vi "Actor Core.vi"(8 "error in":errorcluster, 11 "GObject View in":refnum<class "GObject View.lvclass">) -> (0 "error out":errorcluster, 3 "Actor out":refnum<class "Actor.lvclass">)   [LabVIEW 2013, in "SET Project Editor.lvlib" / "GObject View.lvclass"]
doc: "(<B>Filename</B>: Actor Framework.lvlib:Actor.lvclass:Actor Core.vi)\n\nReceives messages to the actor, reacts to them, and initiates any error handling that may shut the actor down.\n\nDescendant classes may override this VI to append parallel tasks for the actor to complete while it handles messages. Overrides use the Call Parent Method node."
uses:
  GObject View.lvclass
  <vilib>/ActorFramework/Actor/Actor.lvclass
  <vilib>/Utility/miscctls.llb/LVRowAndColumnTypeDef.ctl
  <vilib>/ActorFramework/Actor/Actor.lvclass/Actor.ctl
  <vilib>/ActorFramework/Message Enqueuer/Message Enqueuer.lvclass/Message Enqueuer.ctl
  UI View/UI View.lvclass/UI View.ctl
  MCListbox View Messages/MCLB Request Edit Cell Msg/MCLB Request Edit Cell Msg.lvclass/MCLB Request Edit Cell Msg.ctl
  Controller Messages/Assign Shared Resource Msg/Assign Shared Resource Msg.lvclass/Assign Shared Resource Msg.ctl
  Controller Messages/Remove Object Msg/Remove Object Msg.lvclass/Remove Object Msg.ctl
  MCListbox View/MCListbox View.lvclass/MCListbox View.ctl
  GObject View.lvclass/GObject View.ctl
  MCListbox View/MCListbox View.lvclass
  MCListbox View/Properties/Write Editable From.vi
  UI View/Read UUID.vi
  <vilib>/ActorFramework/Message Enqueuer/Init from Existing Queue.vi
  <vilib>/ActorFramework/Message Enqueuer/Enqueue.vi
  <vilib>/ActorFramework/Message Priority Queue/Priority Enqueue.vi
  <vilib>/ActorFramework/Message Enqueuer/Message Enqueuer.lvclass
  <vilib>/ActorFramework/Stop Msg/Stop Msg.lvclass
  MCListbox View Messages/MCLB Request Edit Cell Msg/MCLB Request Edit Cell Msg.lvclass
  Controller Messages/Assign Shared Resource Msg/Assign Shared Resource Msg.lvclass
  Controller Messages/Remove Object Msg/Remove Object Msg.lvclass
  MCListbox View Messages/MCLB StrEdit Resize Msg/MCLB StrEdit Resize Msg.lvclass
  Lib/Unicode/SET_Unicode Tools.lvlib
panel:
  out "UID":string
  out "ClassName":string
  out "Label":string
  in  "StrEdit":string
  in  "Items":i32(listbox)
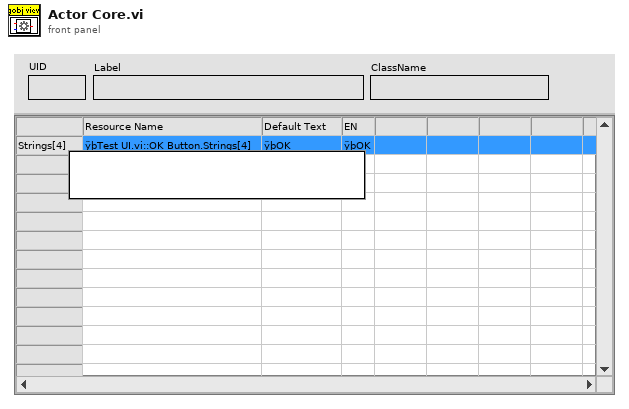
[diagram p1: front panel]
types:
  T1 = typedef "LVRowAndColumnTypeDef.ctl" = cluster{"Row":i32, "Column":i32}
  T2 = typedef "LVPoint32TypeDef.ctl" = cluster{"Horizontal":i32, "Vertical":i32}
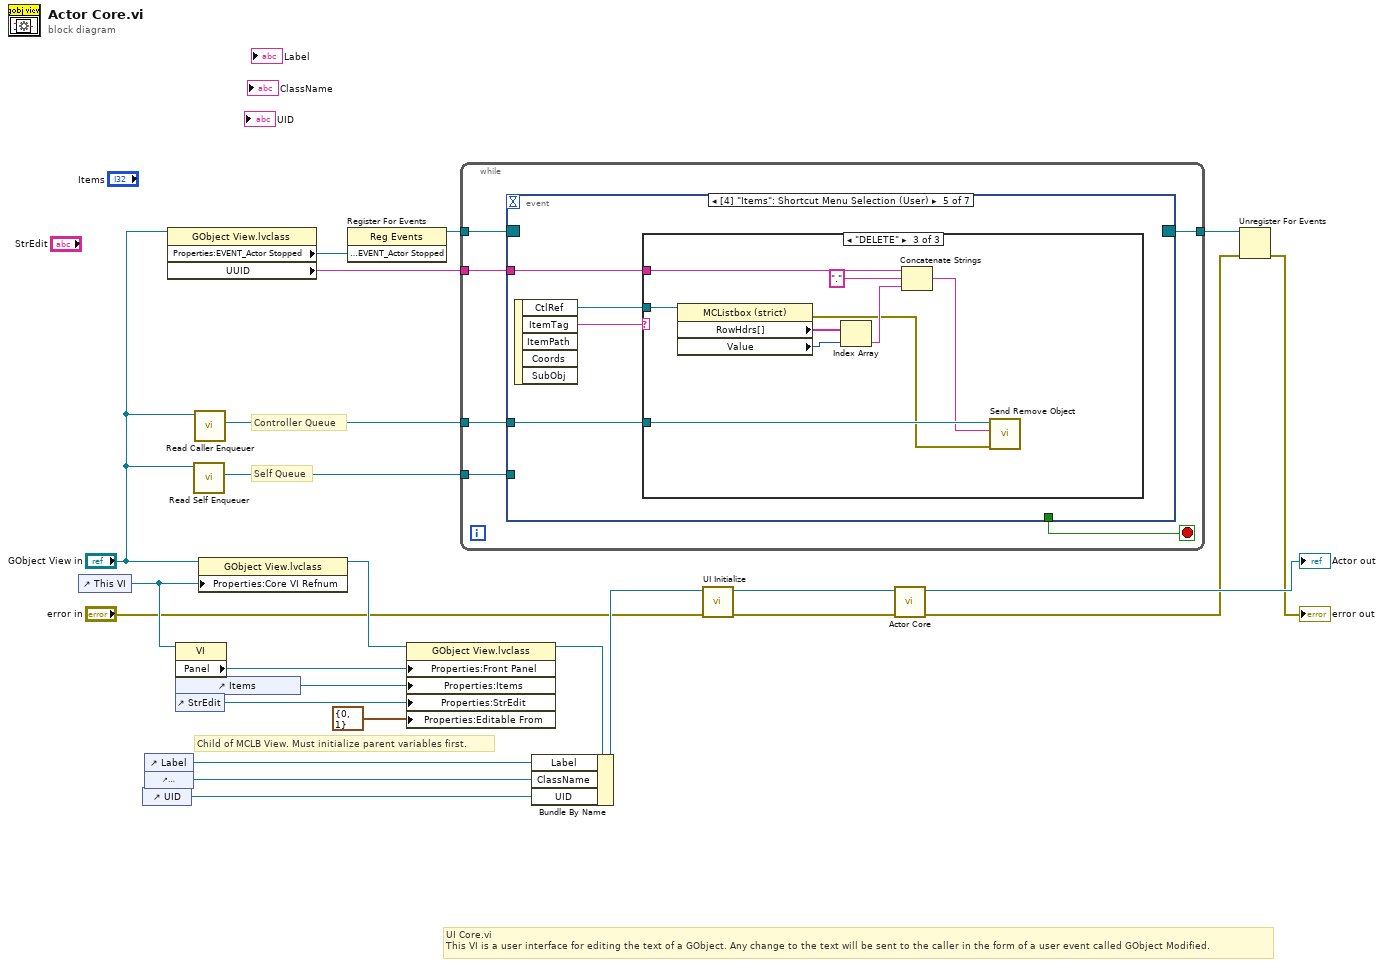
[diagram p0: block diagram]
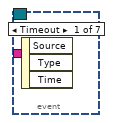
[diagram p2: hidden frame]
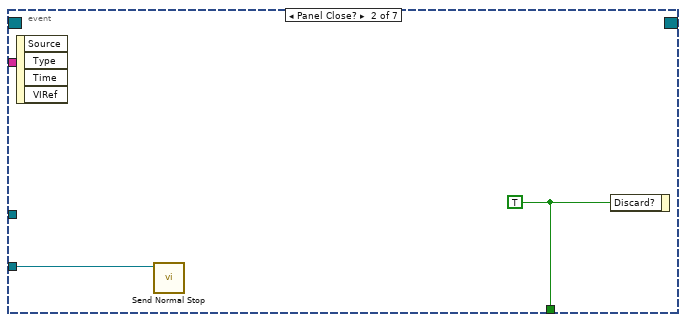
[diagram p3: hidden frame]
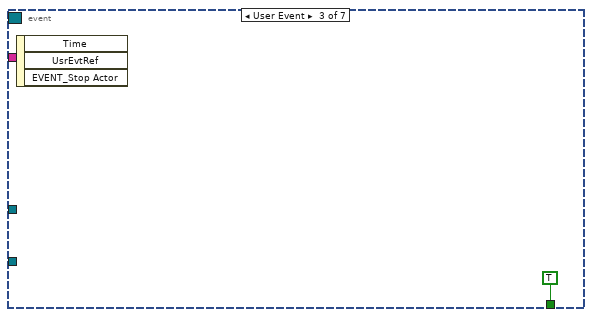
[diagram p4: hidden frame]
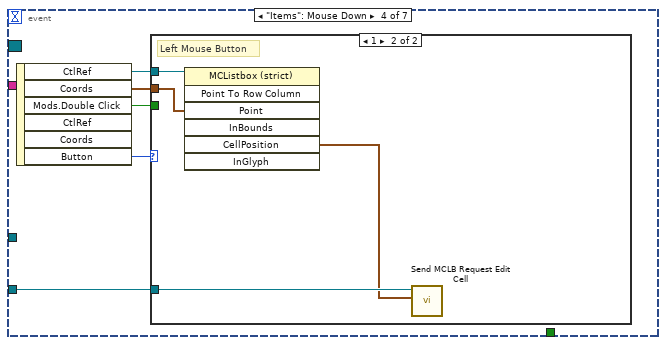
[diagram p5: hidden frame]
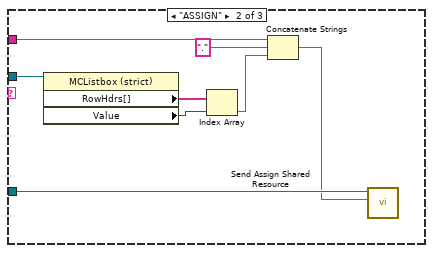
[diagram p8: hidden frame]
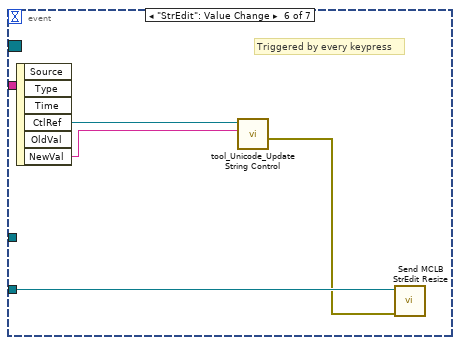
[diagram p9: hidden frame]
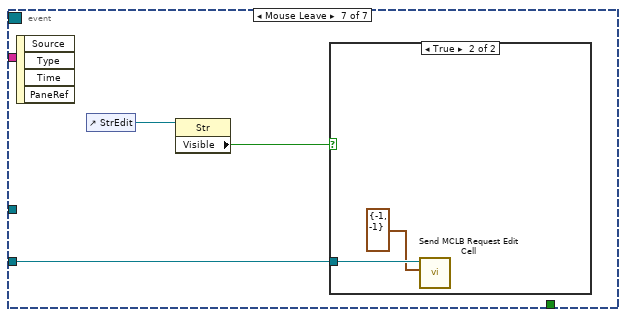
[diagram p10: hidden frame]
diagram:
  # "Child of MCLB View. Must initialize parent variables first."
  # "Controller Queue"
  # "UI Core.vi\nThis VI is a user interface for editing the text of a GObject. Any change to the text will be sent to the caller in the form of a user event called GObject Modified."
  # "Self Queue"
  n1 = control-ref of="This VI"() -> (w16:refnum<vi>)
  n2 = control-ref of="UID"() -> (w13:refnum<vi>)
  n3 = control-ref of="Label"() -> (w15:refnum<vi>)
  n4 = control-ref of="ClassName"() -> (w14:refnum<vi>)
  n5 = property class="GObject View.lvclass"(reference="GObject View in") -> ("Properties:EVENT_Actor Stopped"=w23:refnum<user-event>, "UUID"=w1:string)  [unwired: 1 in, 2 out]
  n6 = property class="VI"(reference=w16) -> ("Panel"=w10:refnum<vi>)  [unwired: 1 in, 2 out]
  n7 = control-ref of="Items"() -> (w9:refnum<vi>)
  n8 = control-ref of="StrEdit"() -> (w8:refnum<vi>)
  n9 = call <vilib>:"Read Self Enqueuer.vi"("Actor"="GObject View in") -> ("Self Enqueuer"=w12:refnum<class "Message Enqueuer.lvclass">)  [unwired: 10 in]
  n10 = call <vilib>:"Read Caller Enqueuer.vi"("Actor"="GObject View in") -> ("Caller Enqueuer"=w18:refnum<class "Message Enqueuer.lvclass">)  [unwired: 10 in]
  n11 = property class="GObject View.lvclass"(reference="GObject View in", "Properties:Core VI Refnum"=w16) -> (reference out=w11:refnum<class "GObject View.lvclass">)  [unwired: 1 in, 1 out]
  n12 = register-events(w23) -> (reference out=w22:refnum<event-registration>)  [unwired: 2 in, 1 out]
  n13 = property class="GObject View.lvclass"(reference=w11, "Properties:Front Panel"=w10, "Properties:Items"=w9, "Properties:StrEdit"=w8, "Properties:Editable From"=T1 {"Row"=0, "Column"=1} ("Editable From")) -> (reference out=w7:refnum<class "GObject View.lvclass">)  [unwired: 1 in, 1 out]
  n14 = while {
    tunnel: w22 -> [w29]
    tunnel: [w28] -> w21
    tunnel: w12 -> [w27]
    tunnel: w18 -> [w26]
    tunnel: w1 -> [w25]
    stop <- w30 stop-if-true
    n15 = event shown="[4] \"Items\": Shortcut Menu Selection (User)" {
      selector: w29 -> [_ _ _ _ _ _ _]
      dyn-events: [_ _ _ _ _ _ _] -> w28
      timeout: _ -> [_ _ _ _ _ _ _]
      tunnel: [_ w32 TRUE ("Discard?") _ _ _ _] -> w30
      tunnel: w27 -> [_ w31 _ w34 _ w65 w68]
      tunnel: w26 -> [_ _ _ _ w45 _ _]
      tunnel: w25 -> [_ _ _ _ w43 _ _]
      event Timeout {
        n16 = event-data() -> ()  [unwired: 1 in, 3 out]
      }
      event Panel Close? {
        w32 = TRUE ("Discard?")
        n17 = event-data() -> ()  [unwired: 1 in, 4 out]
        n18 = call <vilib>:"Send Normal Stop.vi"("Message Enqueuer"=w31) -> ()  [unwired: 10 in, 1 out]
        n19 = event-data("Discard?"=w32) -> ()  [unwired: 1 in, 1 out]
      }
      event User Event {
        n20 = event-data() -> ()  [unwired: 1 in, 3 out]
      }
      event "Items": Mouse Down {
        n21 = event-data() -> ("CtlRef"=w37:refnum<vi>, "Coords"=w36:T2, "Mods.Double Click"=w35:bool, "Button"=w38:u16)  [unwired: 1 in, 2 out]
        n22 = case shown="1" w38 {
          tunnel: w37 -> [_ w42]
          tunnel: w36 -> [_ w41]
          tunnel: w35 -> [_ _]
          tunnel: w34 -> [_ w40]
          frame 0, Default {
          }
          frame 1 {
            # "Left Mouse Button"
            n23 = invoke class="MCListbox (strict)" method="Point To Row Column"(reference=w42, "Point"=w41) -> ("CellPosition"=w39:T1)  [unwired: 5 in, 6 out]
            n24 = call "Send MCLB Request Edit Cell.vi"("RowAndCollumn"=w39, "Message Enqueuer"=w40) -> ()  [unwired: 8 in, 2 out]
          }
        }
      }
      event "Items": Shortcut Menu Selection (User) {
        n25 = event-data() -> ("CtlRef"=w44:refnum<vi>, "ItemTag"=w46:string)  [unwired: 1 in, 3 out]
        n26 = case shown="\"DELETE\"" w46 {
          tunnel: w45 -> [_ w54 w57]
          tunnel: w44 -> [_ w53 w63]
          tunnel: w43 -> [_ w50 w60]
          frame Default {
          }
          frame "ASSIGN" {
            n27 = property class="MCListbox (strict)"(reference=w53) -> ("RowHdrs[]"=w52:string[], "Value"=w51:i32)  [unwired: 1 in, 2 out]
            n28 = Index Array(array=w52, index=w51) -> (element=w48:string)
            n29 = Concatenate Strings(w50, "." ("string"), w48) -> (w47:string)
            n30 = call "Send Assign Shared Resource.vi"("UID"=w47, "Message Enqueuer"=w54) -> ()  [unwired: 8 in, 2 out]
          }
          frame "DELETE" {
            n31 = property class="MCListbox (strict)"(reference=w63) -> (error out=w55:errorcluster, "RowHdrs[]"=w62:string[], "Value"=w61:i32)  [unwired: 1 in, 1 out]
            n32 = Index Array(array=w62, index=w61) -> (element=w58:string)
            n33 = Concatenate Strings(w60, "." ("string"), w58) -> (w56:string)
            n34 = call "Send Remove Object.vi"("error in (no error)"=w55, "UUID"=w56, "Message Enqueuer"=w57) -> ()  [unwired: 7 in, 2 out]
          }
        }
      }
      event "StrEdit": Value Change {
        # "Triggered by every keypress"
        n35 = event-data() -> ("CtlRef"=w67:refnum<vi>, "NewVal"=w66:string)  [unwired: 1 in, 4 out]
        n36 = call "tool_Unicode_Update String Control.vi"("String (UTF-16)"=w66, "*StrControl in"=w67) -> ("error out"=w64:errorcluster)  [unwired: 8 in, 1 out]
        n37 = call "Send MCLB StrEdit Resize.vi"("error in (no error)"=w64, "Message Enqueuer"=w65) -> ()  [unwired: 8 in, 2 out]
      }
      event Mouse Leave {
        n38 = event-data() -> ()  [unwired: 1 in, 4 out]
        n39 = control-ref of="StrEdit"() -> (w70:refnum<vi>)
        n40 = property class="Str"(reference=w70) -> ("Visible"=w69:bool)  [unwired: 1 in, 2 out]
        n41 = case shown="True" w69 {
          tunnel: w68 -> [_ w72]
          frame False {
          }
          frame True {
            n42 = call "Send MCLB Request Edit Cell.vi"("RowAndCollumn"=T1 {"Row"=-1, "Column"=-1} ("Cell Position"), "Message Enqueuer"=w72) -> ()  [unwired: 8 in, 2 out]
          }
        }
      }
    }
  }
  n43 = Bundle By Name(cluster=w7, "Label"=w15, "ClassName"=w14, "UID"=w13) -> (w4:refnum<class "GObject View.lvclass">)
  n44 = call-dynamic "UI Initialize.vi"("error in (no error)"="error in", "GObject View in"=w4) -> ("error out"=w2:errorcluster, "GObject View out"=w5:refnum<class "GObject View.lvclass">)  [unwired: 8 in]
  n45 = call-parent "Actor Core.vi"("error in"=w2, "Actor in"=w5) -> ("error out"=w20:errorcluster, "Actor out"=→"Actor out":refnum<class "Actor.lvclass">)  [unwired: 8 in]
  n46 = Unregister For Events(event registration refnum=w21, error in=w20) -> (error out=→"error out":errorcluster)
